vi "ex1.vi"() -> ()   [LabVIEW 2022 SP3]
uses:
  #typedef_product.ctl
  #typedef_ex1_states.ctl
  #typedef_Program_data.ctl
panel:
  in  "Sort By Creator":string
  in  "Sort By Number":string
  in  "Sort By Name":string
  in  "Sort By Number":bool
  in  "Sort By Name":bool
  in  "Sort By Creator":bool
  in  "Searching Thing":string
  in  "Searching Thing":bool
  in  "Save To File":bool
  in  "Read From File":bool
  in  "Stop Program":bool
  in  "Previous Product":bool
  in  "Next Product":bool
  in  "Remove Product":bool
  in  "Add Product":bool
  out "Product":T1
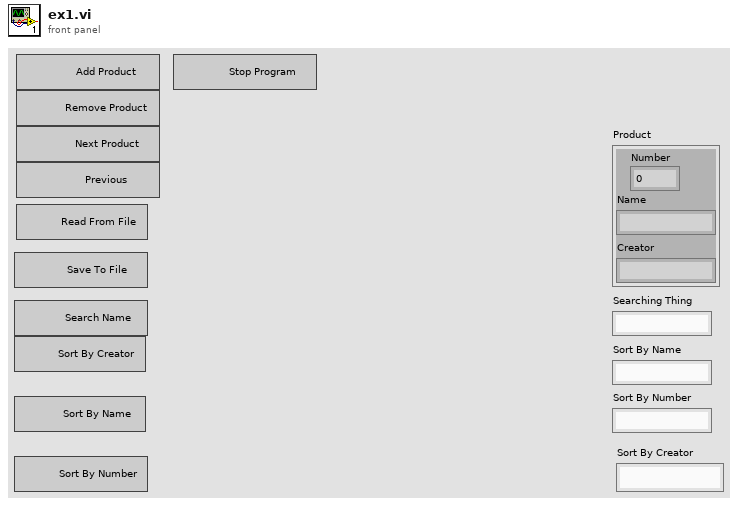
[diagram p1: front panel]
types:
  T1 = typedef "#typedef_product.ctl" = cluster{"Number ":i32, "Name":string, "Creator":string}
  T2 = typedef "#typedef_ex1_states.ctl" = enum16{"Initialize", "Idle", "Add Product", "Remove Student", "Show Next", "Show Prevoius", "Refresh GUI", "Save", "Read", "Searching", "Sort By Name", "Sort By Number", "Sort By Creator", "Error Handler", "Exit"}
  T3 = typedef "#typedef_Program_data.ctl" = cluster{"Products":T1[], "Current Product":i32, "ProductData":path, "Searching thing":string, "Sort By":string}
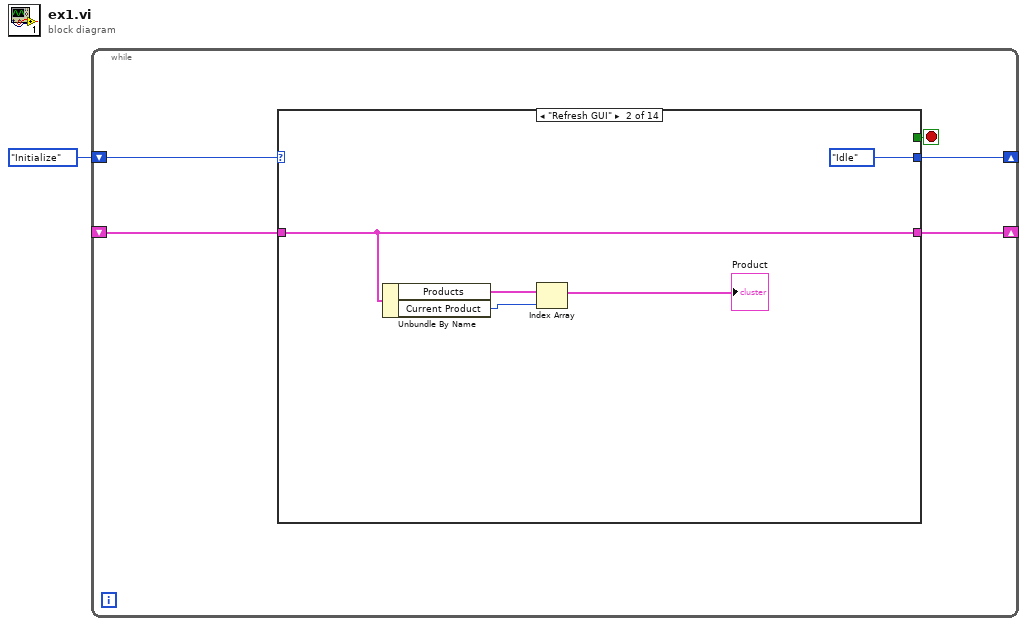
[diagram p0: block diagram]
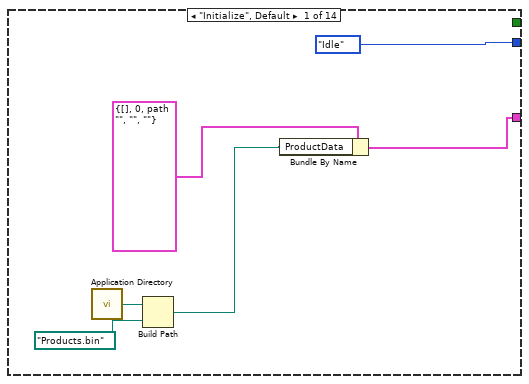
[diagram p2: hidden frame]
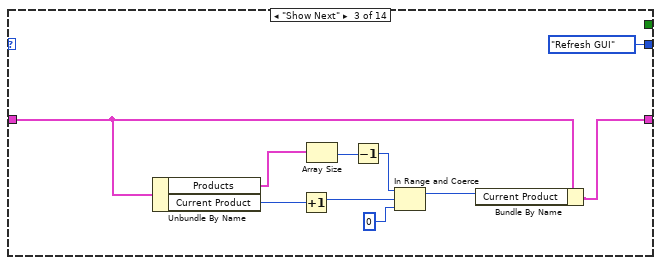
[diagram p3: hidden frame]
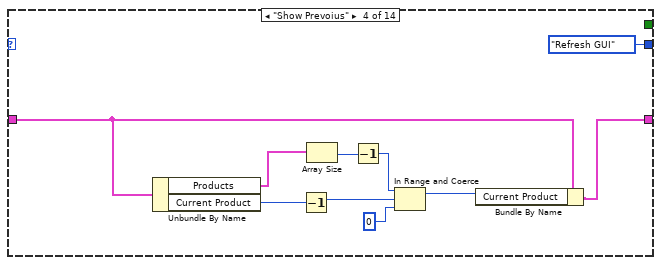
[diagram p4: hidden frame]
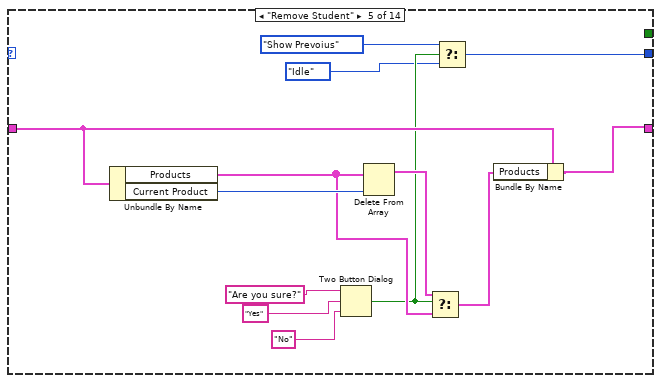
[diagram p5: hidden frame]
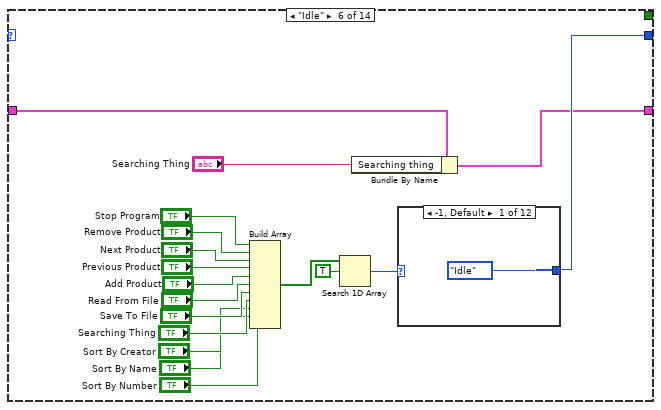
[diagram p6: hidden frame]
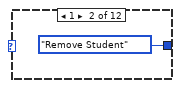
[diagram p7: hidden frame]
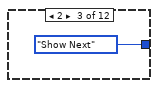
[diagram p8: hidden frame]
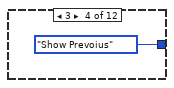
[diagram p9: hidden frame]
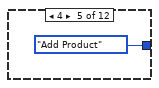
[diagram p10: hidden frame]
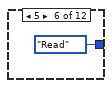
[diagram p11: hidden frame]
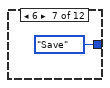
[diagram p12: hidden frame]
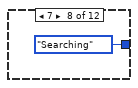
[diagram p13: hidden frame]
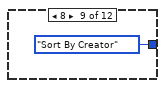
[diagram p14: hidden frame]
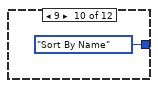
[diagram p15: hidden frame]
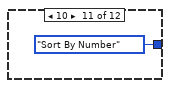
[diagram p16: hidden frame]
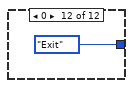
[diagram p17: hidden frame]
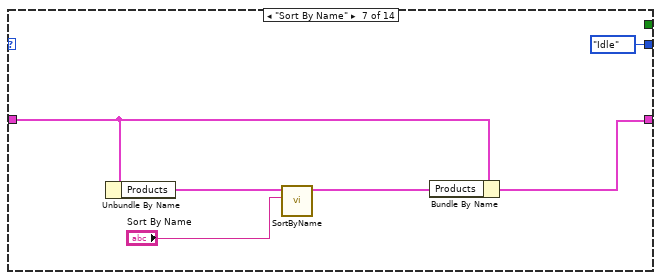
[diagram p18: hidden frame]
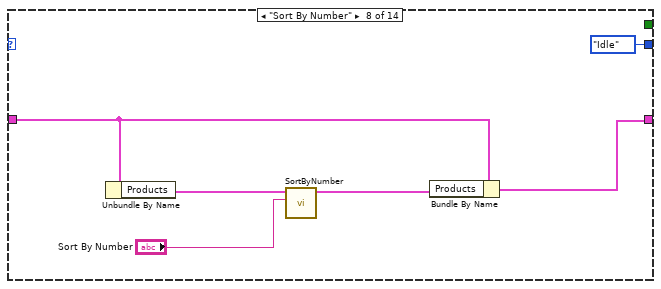
[diagram p19: hidden frame]
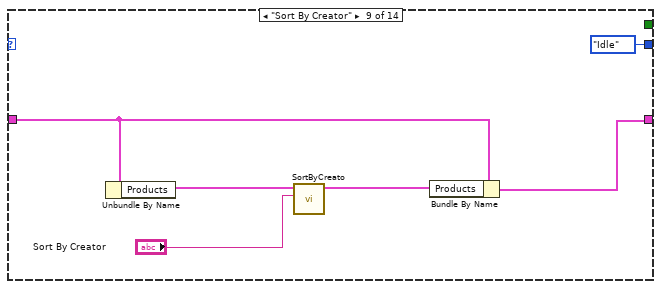
[diagram p20: hidden frame]
diagram:
  n1 = while {
    shift-right: [w5] -> _
    shift-left: #typedef_ex1_states."Initialize" ("SM_States") -> [w6]
    shift-right: [w4] -> _
    shift-left: _ -> [w3]
    stop <- w2 stop-if-true
    n2 = case shown="\"Refresh GUI\"" w6 {
      tunnel: [_ _ _ _ _ _ _ _ _ _ _ _ TRUE _] -> w2
      tunnel: [#typedef_ex1_states."Idle" ("SM_States") #typedef_ex1_states."Idle" ("SM_States") #typedef_ex1_states."Refresh GUI" ("SM_States") #typedef_ex1_states."Refresh GUI" ("SM_States") w38 w60 #typedef_ex1_states."Idle" ("SM_States") #typedef_ex1_states."Idle" ("SM_States") #typedef_ex1_states."Idle" ("SM_States") #typedef_ex1_states."Refresh GUI" ("SM_States") #typedef_ex1_states."Idle" ("SM_States") #typedef_ex1_states."Idle" ("SM_States") #typedef_ex1_states."Exit" ("SM_States") #typedef_ex1_states."Refresh GUI" ("SM_States")] -> w5
      tunnel: [w10 w17 w20 w30 w48 w54 w82 w91 w97 w105 w112 w113 w119 w126] -> w4
      tunnel: w3 -> [_ w17 w22 w32 w50 w55 w83 w92 w98 w106 w112 w116 w119 w127]
      frame "Initialize", Default {
        n3 = call <vilib>:"Application Directory.vi"() -> ("Application Directory"=w9:path)
        n4 = Build Path(base path=w9, name or relative path=path "Products.bin") -> (appended path=w7:path)
        n5 = Bundle By Name(cluster=T3 {"Products"=[], "Current Product"=0, "ProductData"=path "", "Searching thing"="", "Sort By"=""} ("Program Data"), "ProductData"=w7) -> (w10:T3)
      }
      frame "Refresh GUI" {
        n6 = Unbundle By Name(w17) -> ("Products"=w16:T1[], "Current Product"=w13:i32)
        n7 = Index Array(array=w16, index=w13) -> (element=→"Product":T1)
      }
      frame "Show Next" {
        n8 = Unbundle By Name(w22) -> ("Products"=w25:T1[], "Current Product"=w26:i32)
        n9 = Increment(x=w26) -> (x+1=w24:i32)
        n10 = Array Size(array=w25) -> (size(s)=w19:i32)
        n11 = Decrement(x=w19) -> (x-1=w18:i32)
        n12 = In Range and Coerce(upper limit=w18, x=w24, lower limit=0) -> (coerced(x)=w21:i32)  [unwired: 1 out]
        n13 = Bundle By Name(cluster=w22, "Current Product"=w21) -> (w20:T3)
      }
      frame "Show Prevoius" {
        n14 = Unbundle By Name(w32) -> ("Products"=w35:T1[], "Current Product"=w36:i32)
        n15 = Decrement(x=w36) -> (x-1=w34:i32)
        n16 = Array Size(array=w35) -> (size(s)=w29:i32)
        n17 = Decrement(x=w29) -> (x-1=w28:i32)
        n18 = In Range and Coerce(upper limit=w28, x=w34, lower limit=0) -> (coerced(x)=w31:i32)  [unwired: 1 out]
        n19 = Bundle By Name(cluster=w32, "Current Product"=w31) -> (w30:T3)
      }
      frame "Remove Student" {
        n20 = Unbundle By Name(w50) -> ("Products"=w44:T1[], "Current Product"=w49:i32)
        n21 = Two Button Dialog(message="Are you sure?", 1:"No" ("button name (\"OK\")"), 2:"Yes" ("button name (\"OK\")")) -> (T button?=w41:bool)
        n22 = Delete From Array(array=w44, index=w49) -> (array with subset deleted=w43:T1[])  [unwired: 1 in, 1 out]
        n23 = Select(t=w43, s=w41, f=w44) -> (s? t:f=w42:T1[])
        n24 = Select(t=#typedef_ex1_states."Show Prevoius" ("SM_States"), s=w41, f=#typedef_ex1_states."Idle" ("SM_States")) -> (s? t:f=w38:T2)
        n25 = Bundle By Name(cluster=w50, "Products"=w42) -> (w48:T3)
      }
      frame "Idle" {
        n26 = Build Array("Stop Program", "Remove Product", "Next Product", "Previous Product", "Add Product", "Read From File", "Save To File", "Searching Thing", "Sort By Creator", "Sort By Name", "Sort By Number") -> (w63:bool[])
        n27 = Search 1D Array(1D array=w63, element=TRUE) -> (index of element=w61:i32)  [unwired: 1 in]
        n28 = Bundle By Name(cluster=w55, "Searching thing"="Searching Thing") -> (w54:T3)
        n29 = case shown="-1, Default" w61 {
          tunnel: [#typedef_ex1_states."Idle" ("SM_States") #typedef_ex1_states."Remove Student" ("SM_States") #typedef_ex1_states."Show Next" ("SM_States") #typedef_ex1_states."Show Prevoius" ("SM_States") #typedef_ex1_states."Add Product" ("SM_States") #typedef_ex1_states."Read" ("SM_States") #typedef_ex1_states."Save" ("SM_States") #typedef_ex1_states."Searching" ("SM_States") #typedef_ex1_states."Sort By Creator" ("SM_States") #typedef_ex1_states."Sort By Name" ("SM_States") #typedef_ex1_states."Sort By Number" ("SM_States") #typedef_ex1_states."Exit" ("SM_States")] -> w60
          frame -1, Default {
          }
          frame 1 {
          }
          frame 2 {
          }
          frame 3 {
          }
          frame 4 {
          }
          frame 5 {
          }
          frame 6 {
          }
          frame 7 {
          }
          frame 8 {
          }
          frame 9 {
          }
          frame 10 {
          }
          frame 0 {
          }
        }
      }
      frame "Sort By Name" {
        n30 = Unbundle By Name(w83) -> ("Products"=w86:T1[])
        n31 = call "SortByName.vi"("Sort by"="Sort By Name", "Products"=w86) -> ("Sorted Products"=w84:T1[])  [unwired: 8 in, 1 out]
        n32 = Bundle By Name(cluster=w83, "Products"=w84) -> (w82:T3)
      }
      frame "Sort By Number" {
        n33 = Unbundle By Name(w92) -> ("Products"=w90:T1[])
        n34 = call "SortByNumber.vi"("Sort by"="Sort By Number", "Products"=w90) -> ("Sorted Products"=w88:T1[])  [unwired: 8 in, 1 out]
        n35 = Bundle By Name(cluster=w92, "Products"=w88) -> (w91:T3)
      }
      frame "Sort By Creator" {
        n36 = Unbundle By Name(w98) -> ("Products"=w96:T1[])
        n37 = call "SortByCreato.vi"("Sort by"="Sort By Creator", "Products"=w96) -> ("Sorted Products"=w94:T1[])  [unwired: 8 in, 1 out]
        n38 = Bundle By Name(cluster=w98, "Products"=w94) -> (w97:T3)
      }
      frame "Searching" {
        n39 = Unbundle By Name(w106) -> ("Current Product"=w104:i32, "Products"=w108:T1[], "Searching thing"=w107:string)
        n40 = call "SearchingThings.vi"("Searching thing"=w107, "Products"=w108) -> ("Index of Searching Thing"=w103:i32)  [unwired: 8 in, 1 out]
        n41 = Equal?(x=w103, y=-1) -> (x = y?=w101:bool)
        n42 = Select(t=w104, s=w101, f=w103) -> (s? t:f=w100:i32)
        n43 = Bundle By Name(cluster=w106, "Current Product"=w100) -> (w105:T3)
      }
      frame "Save" {
        n44 = Unbundle By Name(w112) -> ("ProductData"=w110:path, "Products"=w111:T1[])
        n45 = Write to Binary File(file (use dialog)=w110, data=w111) -> ()  [unwired: 4 in, 3 out]
      }
      frame "Read" {
        n46 = Unbundle By Name(w116) -> ("Products"=w114:T1[], "ProductData"=w118:path)
        n47 = Read from Binary File(5:w114, 11:w118) -> (2:w117:T1[])  [unwired: 4 in, 3 out]
        n48 = Bundle By Name(cluster=w116, "Products"=w117) -> (w113:T3)
      }
      frame "Exit" {
        n49 = Unbundle By Name(w119) -> ("ProductData"=w120:path, "Products"=w121:T1[])
        n50 = Write to Binary File(file (use dialog)=w120, data=w121) -> ()  [unwired: 4 in, 3 out]
      }
      frame "Add Product" {
        n51 = call "NewProductDialog.vi"() -> ("Cancelled?"=w124:bool, "NewProduct"=w128:T1)  [unwired: 9 in, 1 out]
        n52 = case shown="False" w124 {
          tunnel: w128 -> [_ w133]
          tunnel: w127 -> [w129 w132]
          tunnel: [w129 w130] -> w126
          frame True {
          }
          frame False {
            n53 = Unbundle By Name(w132) -> ("Products"=w134:T1[])
            n54 = Build Array (concatenate)(w134, w133) -> (w131:T1[])
            n55 = Bundle By Name(cluster=w132, "Products"=w131) -> (w130:T3)
          }
        }
      }
    }
  }
